vi "setUp.vi"(8 "error in (no error)":errorcluster, 11 "reference in":refnum<class "CAN Outgoing Tests.lvclass">) -> (0 "error out":errorcluster, 3 "reference out":refnum<class "CAN Outgoing Tests.lvclass">)   [LabVIEW 2017, in "CAN Outgoing Tests.lvclass"]
doc: "setUp runs prior to the test method during test execution. Use this method to initialize any object data required by your tests."
uses:
  CAN Outgoing Tests.lvclass
  C:/Program Files (x86)/National Instruments/LabVIEW 2017/vi.lib/addons/_JKI Toolkits/VI Tester/TestCase.llb/TestCase.lvclass
  CAN Outgoing Tests.lvclass/CAN Outgoing Tests.ctl
  <vilib>/xnet/xnet.llb/XNET String To IO Name (Frame).vi
  <vilib>/xnet/xnet.llb/XNET String To IO Name (Interface).vi
  <vilib>/xnet/xnet.llb/XNET Create Session (Frame Input Queued).vi
  <vilib>/addons/_JKI Toolkits/VI Tester/TestCase.llb/TestCase.lvclass
  <resource>/objmgr/xnet.rc
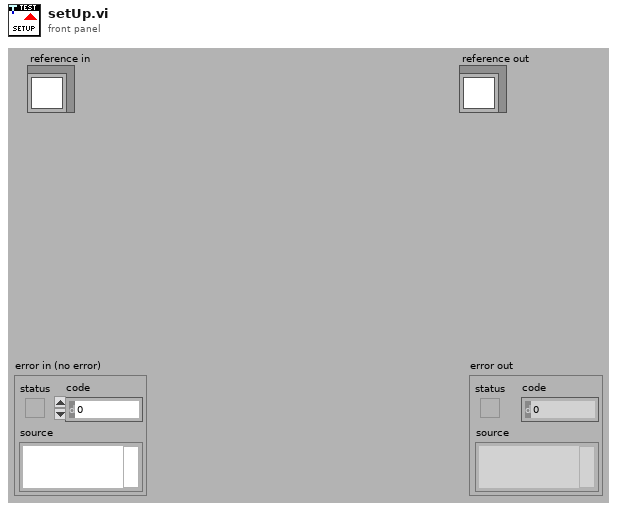
[diagram p1: front panel]
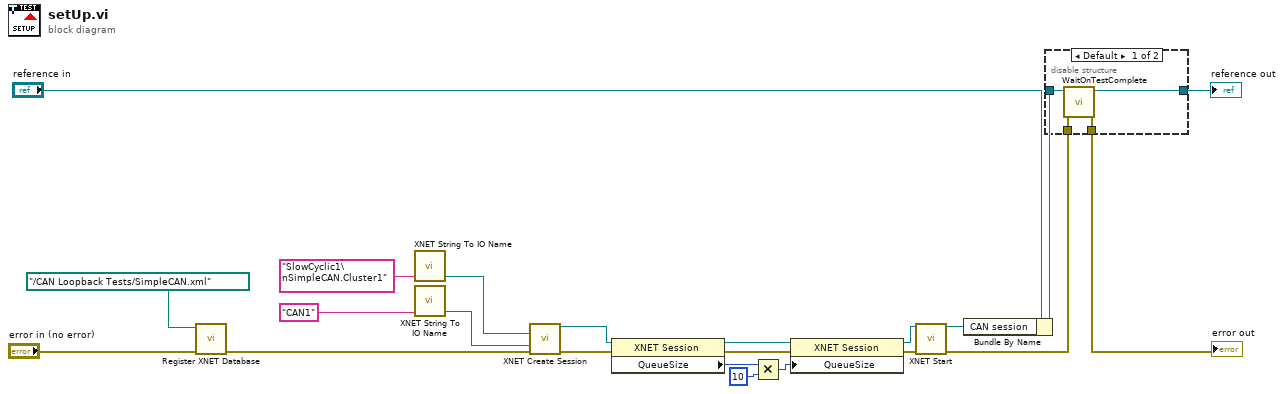
[diagram p0: block diagram]
diagram:
  n1 = call "Register XNET Database.vi"("error in (no error)"="error in (no error)", "database path"=path "../CAN Loopback Tests/SimpleCAN.xml") -> ("error out"=w2:errorcluster)  [unwired: 8 in, 1 out]
  n2 = call-poly <vilib>:"XNET String To IO Name.vi"("string"="SlowCyclic1\nSimpleCAN.Cluster1") -> ("XNET Frame"=w17:refnum<k21>)  [unwired: 4 out]
  n3 = call-poly <vilib>:"XNET String To IO Name.vi"("string"="CAN1") -> ("XNET Interface"=w7:refnum<k21>)  [unwired: 4 out]
  n4 = call-poly <vilib>:"XNET Create Session.vi"("frame"=w17, "interface"=w7, "error in (no error)"=w2) -> ("session out"=w16:refnum<k21>, "error out"=w15:errorcluster)  [unwired: 11 in]
  n5 = property class="XNET Session"(reference=w16, error in=w15) -> (reference out=w14:refnum<k21>, error out=w13:errorcluster, "QueueSize"=w11:u32)
  n6 = Multiply(x=w11, y=u32 10) -> (x*y=w10:u32)
  n7 = property class="XNET Session"(reference=w14, error in=w13, "QueueSize"=w10) -> (reference out=w5:refnum<k21>, error out=w12:errorcluster)
  n8 = call <vilib>:"XNET Start.vi"("session in"=w5, "error in (no error)"=w12) -> ("session out"=w4:refnum<k21>, "error out"=w6:errorcluster)  [unwired: 12 in]
  n9 = Bundle By Name(cluster="reference in", "CAN session"=w4) -> (w19:refnum<class "CAN Outgoing Tests.lvclass">)
  n10 = disable-structure shown="Default" {
    disable-tunnel: w6 -> [w26 w27]
    disable-tunnel: [w25 w27] -> w22
    disable-tunnel: [w24 w28] -> w20
    disable-tunnel: w19 -> [w23 w28]
    frame condition #0 (active) {
      n11 = call <vilib>:"WaitOnTestComplete.vi"("error in (no error)"=w26, "TestCase in"=w23) -> ("error out"=w25:errorcluster, "TestCase out"=w24:refnum<class "CAN Outgoing Tests.lvclass">)  [unwired: 8 in]
    }
    frame condition #1 {
    }
  }
  "error out" <- w22
  "reference out" <- w20
